vi "CPU Temperature.vi"(8 "error in (no error)":errorcluster, 11 "RP Communicator in":refnum<class "RP Communicator VISA.lvclass">) -> (0 "error out":errorcluster, 2 "CPU Temperature":dbl, 3 "RP Communicator out":refnum<class "RP Communicator VISA.lvclass">)   [LabVIEW 2016, in "RP Communicator VISA.lvclass"]
uses:
  RP Communicator VISA.lvclass
  RP Communicator VISA.lvclass/RP Communicator VISA.ctl
  RP Read Temperature VISA.vi
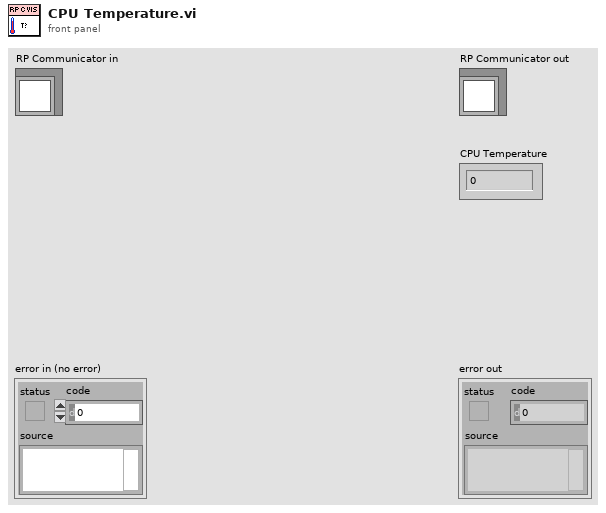
[diagram p1: front panel]
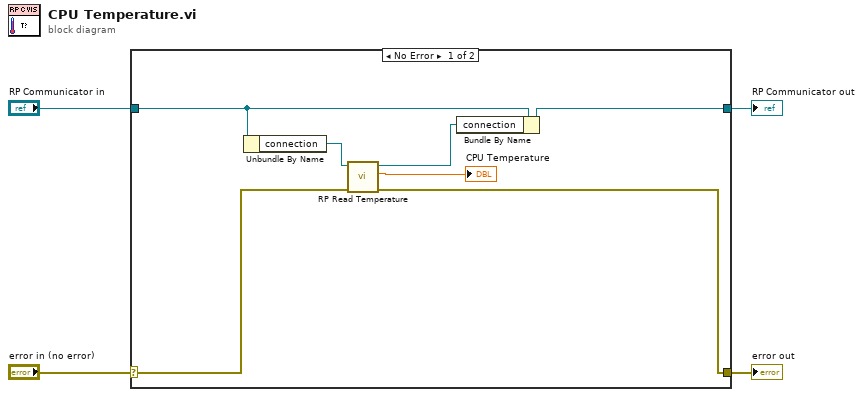
[diagram p0: block diagram]
diagram:
  n1 = case shown="No Error" "error in (no error)" {
    selector: "error in (no error)" -> [w9 w13]
    tunnel: [w8 w13] -> w3
    tunnel: [w7 w12] -> w1
    tunnel: "RP Communicator in" -> [w11 w12]
    frame No Error {
      n2 = Unbundle By Name(w11) -> ("connection"=w10:refnum<visa-resource-name>)
      n3 = call-poly "RP Read Temperature.vi"("Error In"=w9, "VISA resource"=w10) -> ("error out"=w8:errorcluster, "Thermometer"=→"CPU Temperature":dbl, "VISA resource out"=w6:refnum<visa-resource-name>)  [unwired: 7 in]
      n4 = Bundle By Name(cluster=w11, "connection"=w6) -> (w7:refnum<class "RP Communicator VISA.lvclass">)
    }
    frame Error {
    }
  }
  "error out" <- w3
  "RP Communicator out" <- w1
